vi "Camera Get.vi"(1 "Wanted Y Angle":dbl, 2 "Wanted X Angle":dbl) -> ()   [LabVIEW 2013]
uses:
  Camera Global.vi
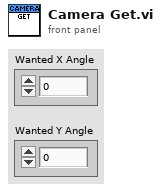
[diagram p1: front panel]
types:
  T1 = cluster{"Manual X Angle":dbl, "Manual Y Angle ":dbl, "Set X Angle":dbl, "Set Y Angle ":dbl, "Wanted X Angle":dbl, "Wanted Y Angle  ":dbl}
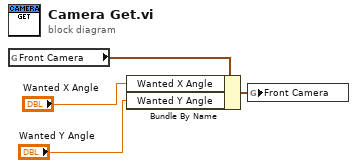
[diagram p0: block diagram]
diagram:
  n1 = global read "Camera Global.vi" "Front Camera"() -> (w3:T1)
  n2 = Bundle By Name(cluster=w3, "Wanted X Angle"="Wanted X Angle", "Wanted Y Angle"="Wanted Y Angle") -> (w4:T1)
  n3 = global write "Camera Global.vi" "Front Camera"(w4) -> ()
